vi "TDMS_ListName.vi"() -> ()   [LabVIEW 2011]
panel:
  out "group names":string[](array[string])
  out "group/channel names":string[][](array[string])
  out "channel":string[][](array[string])
  out "error out":errorcluster
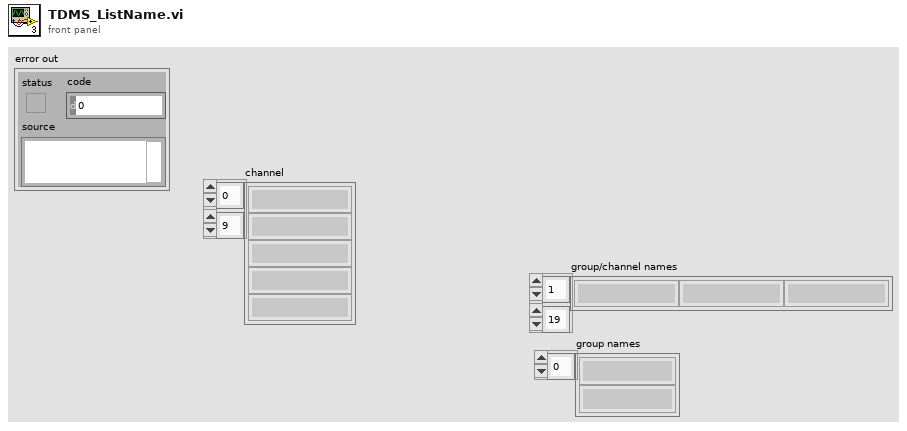
[diagram p1: front panel]
types:
  T1 = enum16{"open", "open or create", "create or replace", "create", "open (read-only)"}
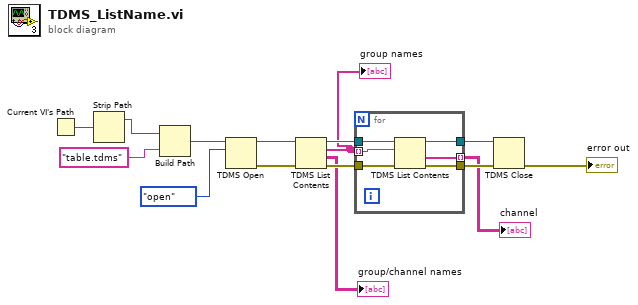
[diagram p0: block diagram]
diagram:
  n1 = Current VI's Path() -> (path=w15:path)
  n2 = Strip Path(path=w15) -> (stripped path=w14:path)  [unwired: 1 out]
  n3 = Build Path(base path=w14, name or relative path="table.tdms") -> (appended path=w11:path)
  n4 = TDMS Open(10:T1."open" ("operation (0:open)"), 11:w11) -> (0:w9:errorcluster, 3:w10:refnum<k34>)  [unwired: 4 in]
  n5 = TDMS List Contents(4:w9, 7:w10) -> (0:w7:errorcluster, 1:→"group/channel names":string[][], 2:w4:string[], 3:w8:refnum<k34>)  [unwired: 1 in]
  "group names" <- w4
  n6 = for {
    tunnel: w8 -> [w21]
    tunnel: w7 -> [w20]
    tunnel: [w19] -> w6
    tunnel: [w18] -> w5
    tunnel: w4 -> [w17] mode=indexing
    tunnel: [w16] -> w3 mode=indexing
    n7 = TDMS List Contents(4:w20, 6:w17, 7:w21) -> (0:w19:errorcluster, 1:w16:string[], 3:w18:refnum<k34>)  [unwired: 1 out]
  }
  "channel" <- w3
  n8 = TDMS Close(8:w6, 11:w5) -> (0:→"error out":errorcluster)  [unwired: 1 out]
